vi "Olivia_TrainerLabVIEW.vi"() -> ()   [LabVIEW 2021]
uses:
  <vilib>/Instr/_visa.llb/VISA Configure Serial Port (Instr).vi
panel:
  out "x/y":dbl
  out "Training String":string
  out "Upload String":string
  in  "Training Data":bool
  in  "Upload":bool
  out "Light Intensity %":dbl(slide) scale=0.0..100.0
  in  "Motor Position":dbl(knob) scale=0.0..180.0 scale format="%^#_3g"
  out "Meter":dbl(knob) scale=0.0..10.0
  out "Status indicator":bool
  out "Boolean 2":bool
  out "Boolean":bool
  out "concatenated string":string
  out "Numeric":i32
  out "return count 3":u32
  out "return count 2":u32
  out "read buffer":string
  out "return count":u32
  out "Motor":string
  out "Sensor":string
  out "Type":string
  out "Name":string
  out "read buffer 3":string
  out "Serial Settings:Number of Bytes at Serial Port 2":u32
  out "read buffer 2":string
  in  "VISA resource name 2":refnum<visa-resource-name>
  out "Value":dbl
  out "Motor":dbl(slide) scale=0.0..180.0
  in  "Done":bool
  in  "Train":bool
  # "View & Train"
  # "Green button that says connected"
  # "help button pops up a help message"
  # "big button to connect - Green light to indicate connection"
  # "move the LED to the top to show connection"
  # "Connect"
  # "Make it go back to this screen when nothing is connected"
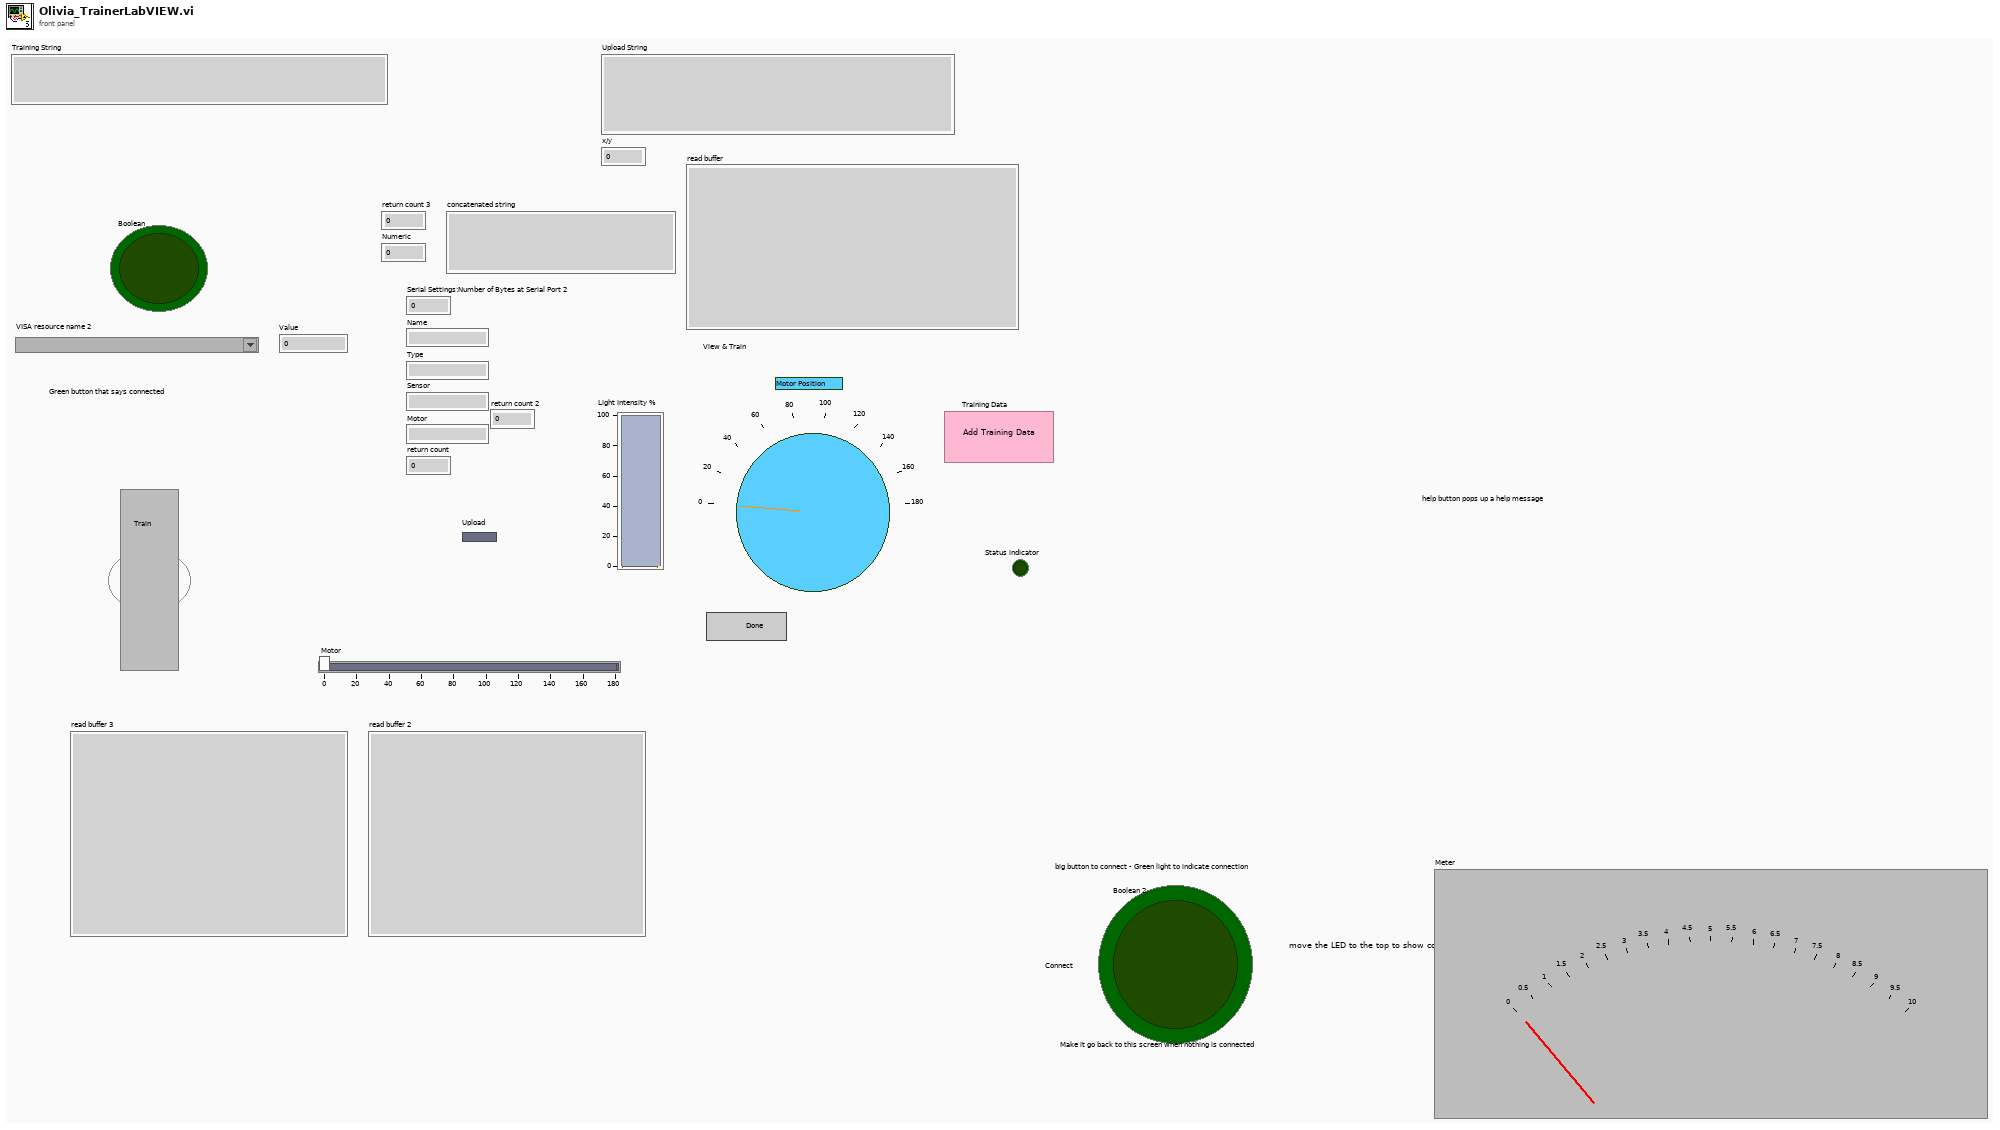
[diagram p1: front panel]
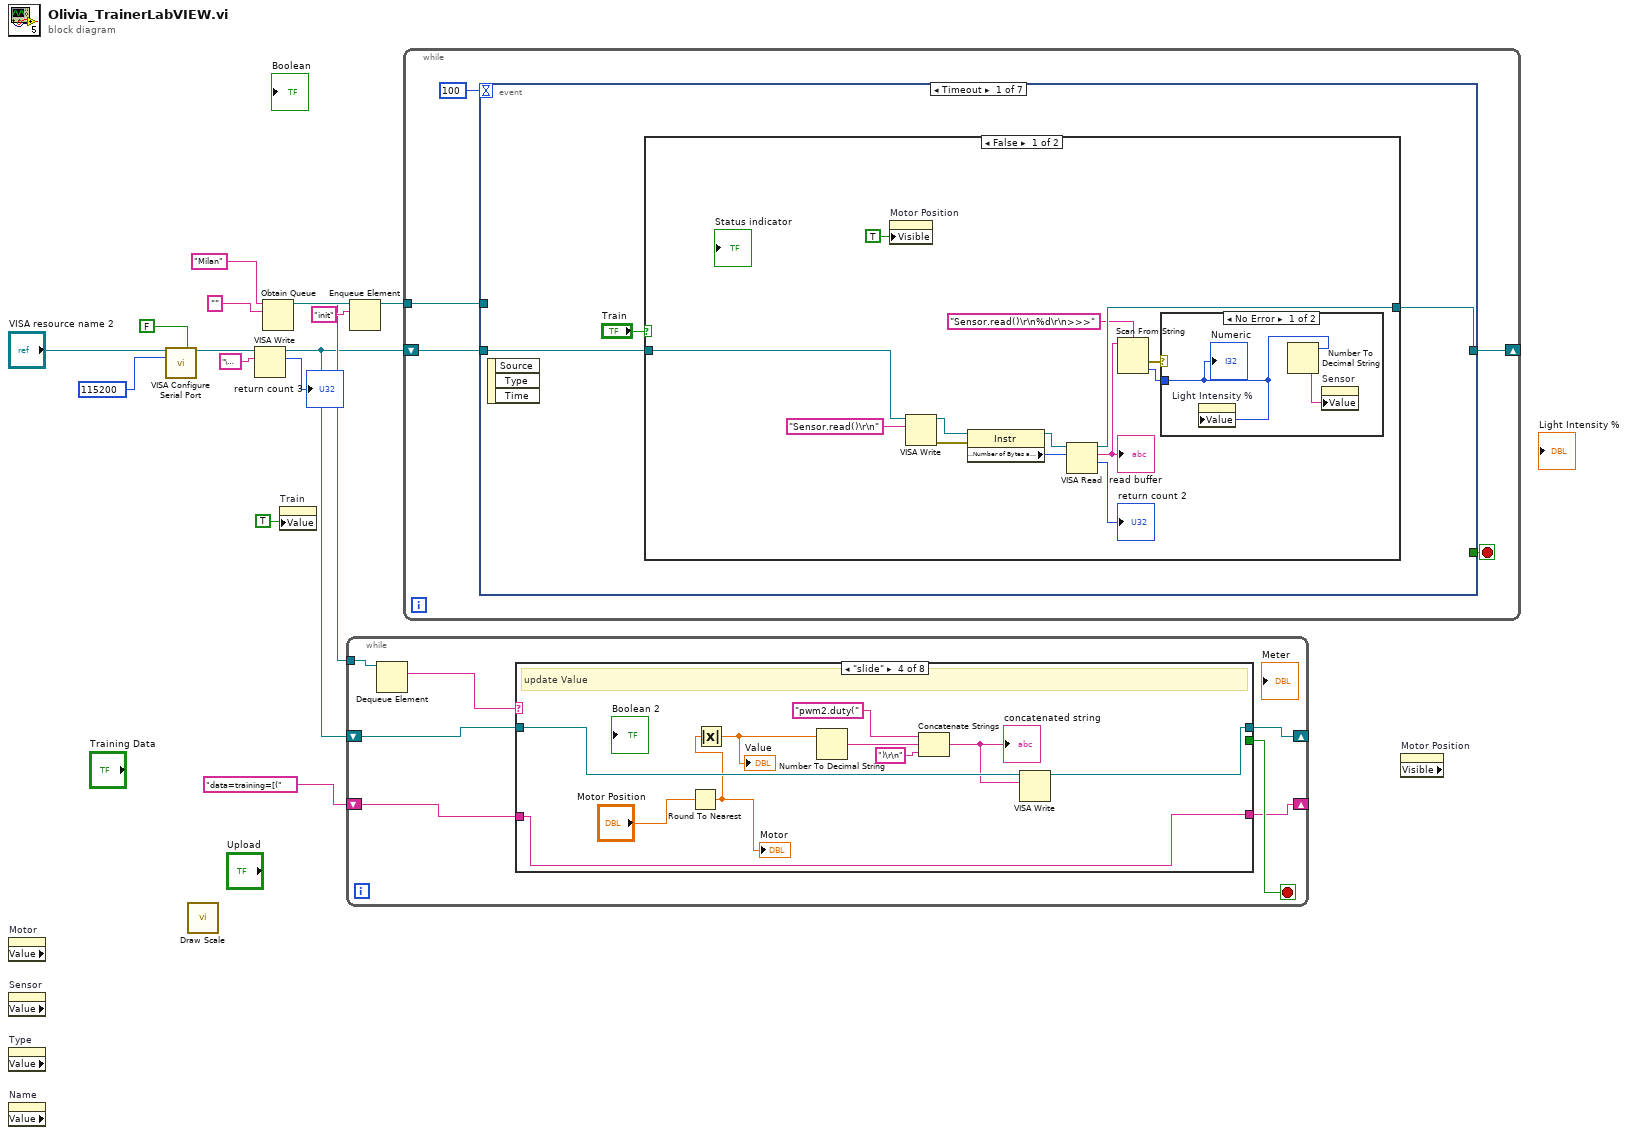
[diagram p0: block diagram]
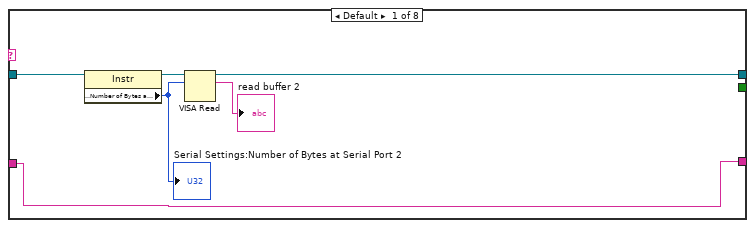
[diagram p2: hidden frame]
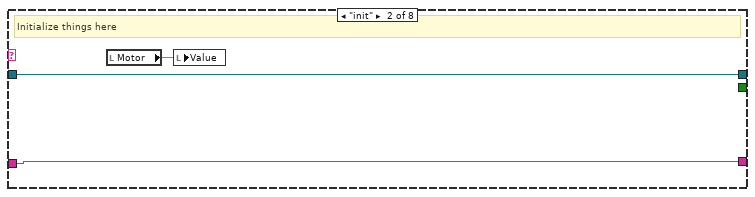
[diagram p3: hidden frame]
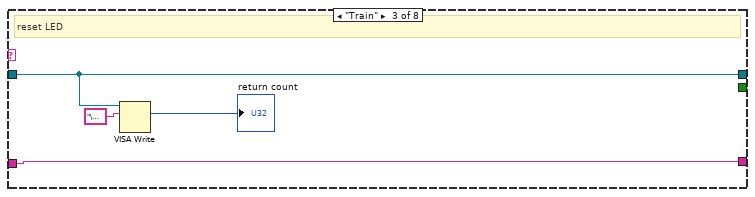
[diagram p4: hidden frame]
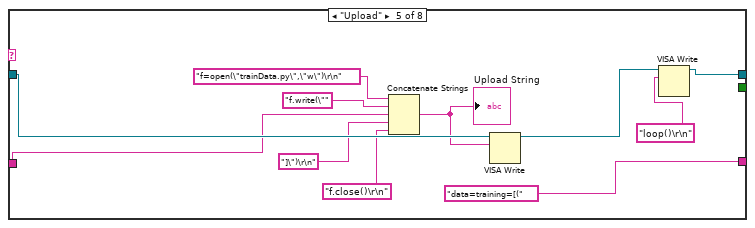
[diagram p5: hidden frame]
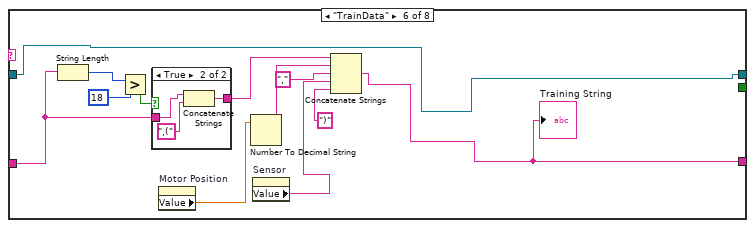
[diagram p6: hidden frame]
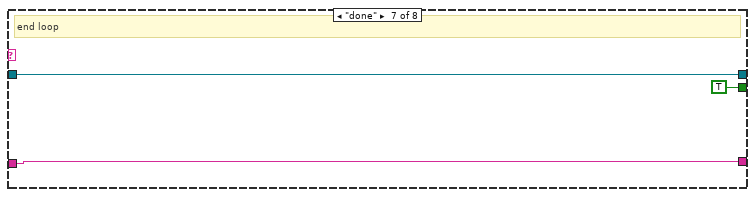
[diagram p8: hidden frame]
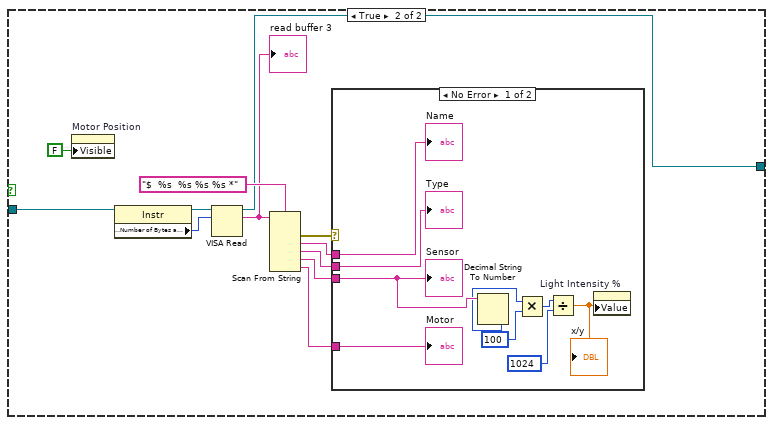
[diagram p11: hidden frame]
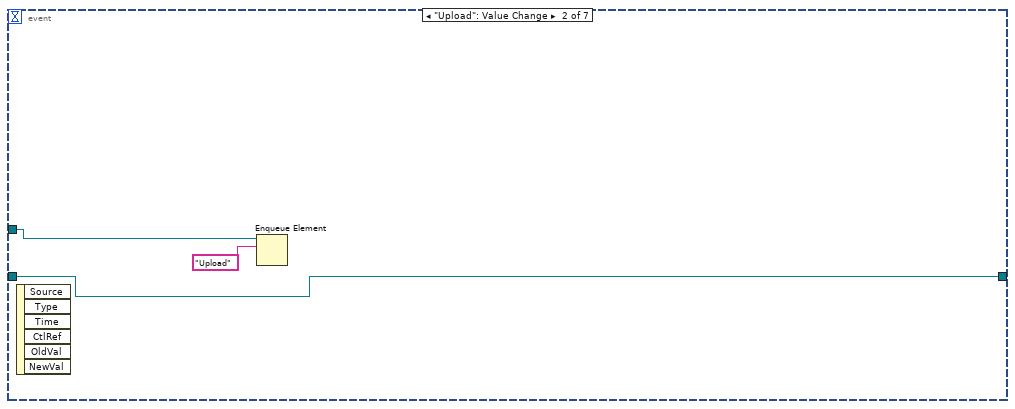
[diagram p13: hidden frame]
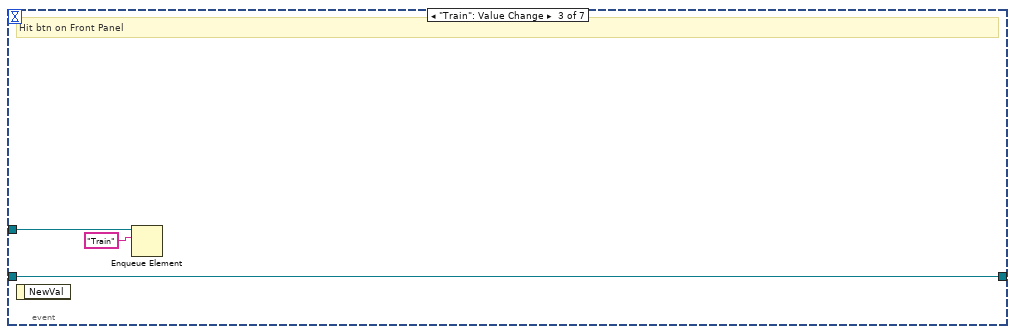
[diagram p14: hidden frame]
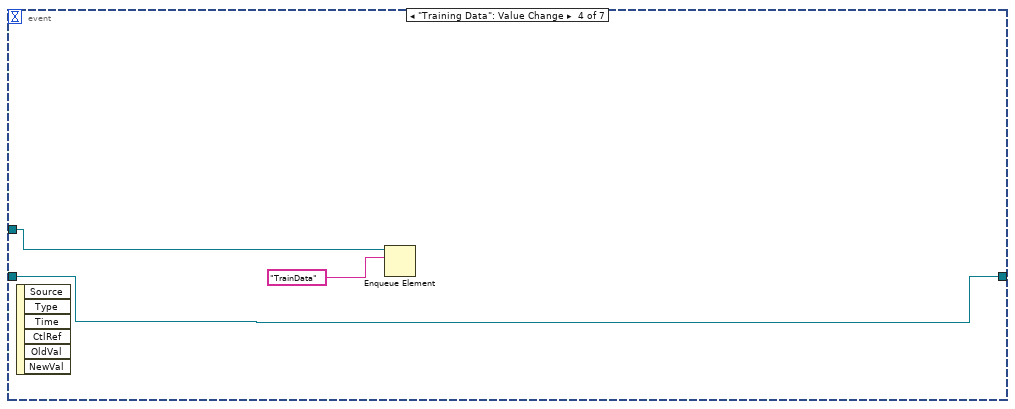
[diagram p15: hidden frame]
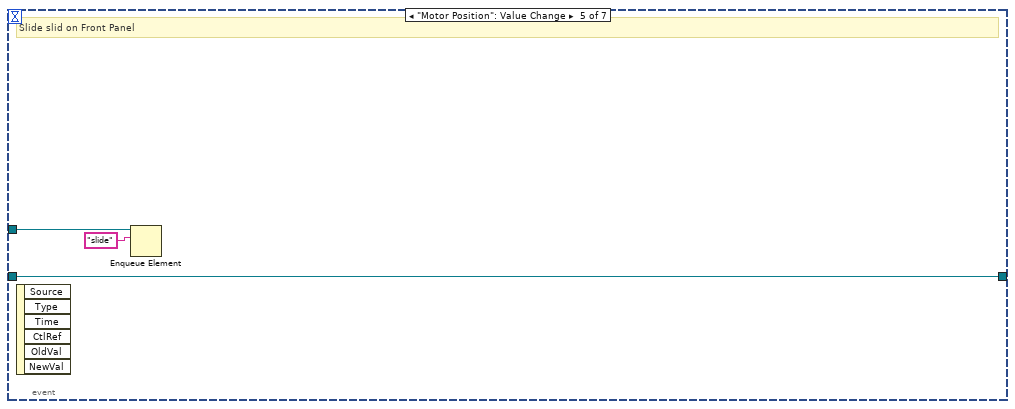
[diagram p16: hidden frame]
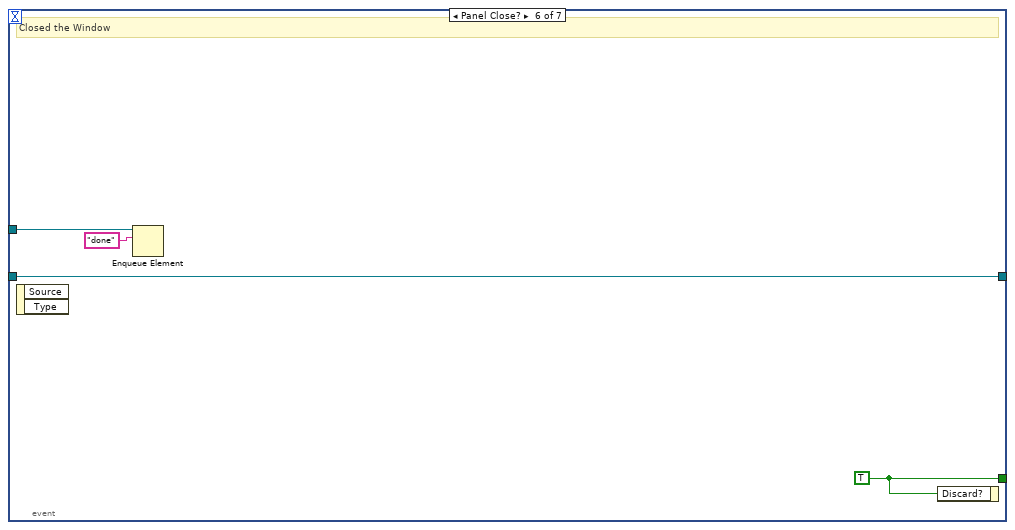
[diagram p17: hidden frame]
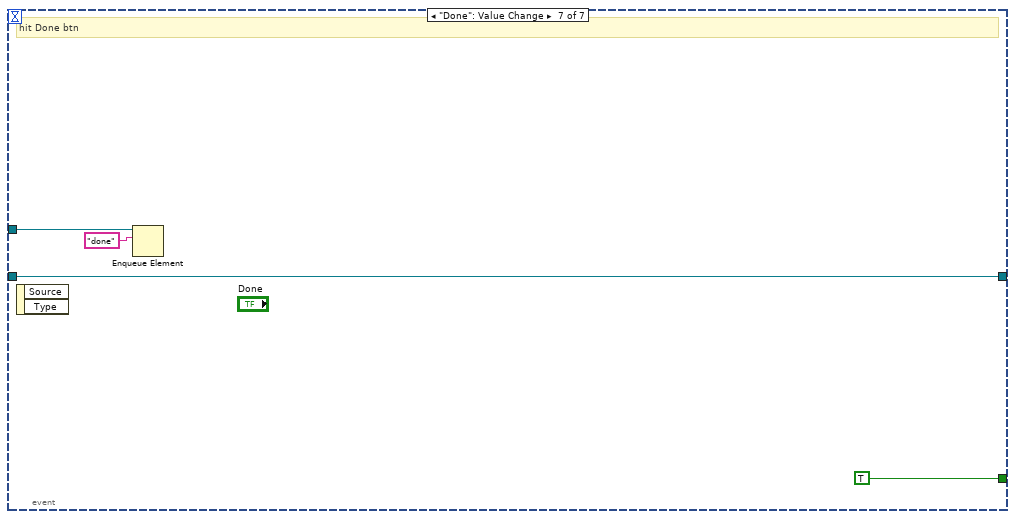
[diagram p18: hidden frame]
diagram:
  n1 = property on="Motor" class="Str" props=["Value"]() -> ()  [unwired: 2 in, 3 out]
  n2 = property on="Sensor" class="Str" props=["Value"]() -> ()  [unwired: 2 in, 3 out]
  n3 = property on="Type" class="Str" props=["Value"]() -> ()  [unwired: 2 in, 3 out]
  n4 = property on="Name" class="Str" props=["Value"]() -> ()  [unwired: 2 in, 3 out]
  n5 = call-poly "VISA Configure Serial Port"("VISA resource name"="VISA resource name 2", "Enable Termination\nChar (T)"=FALSE ("Enable Termination\nChar (T)"), "baud rate (9600)"=u32 115200) -> ("VISA resource name out"=w6:refnum<visa-resource-name>)  [unwired: 11 in, 1 out]
  n6 = call <vilib>:"Draw Scale.vi"() -> ()  [unwired: 11 in, 1 out]
  n7 = VISA Write(VISA resource name=w6, write buffer="\u0004") -> (VISA resource name out=w4:refnum<visa-resource-name>, return count=→"return count 3":u32)  [unwired: 1 in, 1 out]
  n8 = Obtain Queue(name (unnamed)="Milan", element data type="") -> (queue out=w14:refnum<queue>)  [unwired: 3 in, 2 out]
  n9 = property on="Train" class="Bool (strict)"("Value"=TRUE ("Train")) -> ()  [unwired: 2 in, 2 out]
  n10 = Enqueue Element(queue=w14, element="init") -> (queue out=w10:refnum<queue>)  [unwired: 2 in, 2 out]
  n11 = while {
    tunnel: w10 -> [w21]
    shift-right: [w17] -> _
    shift-left: w4 -> [w18]
    shift-right: [w15] -> _
    shift-left: "data=training=[(" -> [w16]
    stop <- w19 stop-if-true
    n12 = Dequeue Element(queue=w21) -> (element=w20:string)  [unwired: 2 in, 3 out]
    n13 = case shown="\"slide\"" w20 {
      tunnel: [_ _ _ _ _ _ TRUE ("Discard?") _] -> w19
      tunnel: w18 -> [w24 w29 w34 w44 w55 w63 w73 w76]
      tunnel: [w23 w29 w34 w39 w46 w63 w73 w76] -> w17
      tunnel: w16 -> [w22 w28 w31 w35 w52 w58 w72 w75]
      tunnel: [w22 w28 w31 w35 "data=training=[(" w56 w72 w75] -> w15
      frame Default {
        n14 = property class="Instr"(reference=w24) -> (reference out=w25:refnum<visa-resource-name>, "Serial Settings:Number of Bytes at Serial Port"=w26:u32)  [unwired: 1 in, 1 out]
        "Serial Settings:Number of Bytes at Serial Port 2" <- w26
        n15 = VISA Read(VISA resource name=w25, byte count=w26) -> (VISA resource name out=w23:refnum<visa-resource-name>, read buffer=→"read buffer 2":string)  [unwired: 1 in, 2 out]
      }
      frame "init" {
        # "Initialize things here"
        n16 = local read "Motor"() -> (w30:dbl)
        n17 = local write "Value"(w30) -> ()
      }
      frame "Train" {
        # "reset LED"
        n18 = VISA Write(VISA resource name=w34, write buffer="\u0003") -> (return count=→"return count":u32)  [unwired: 1 in, 2 out]
      }
      frame "slide" {
        # "update Value"
        n19 = Round To Nearest(number="Motor Position") -> (nearest integer value=w36:dbl)
        "Motor" <- w36
        n20 = Absolute Value(x=w36) -> (abs(x)=w38:dbl)
        "Value" <- w38
        n21 = Number To Decimal String(number=w38) -> (decimal integer string=w42:string)  [unwired: 1 in]
        n22 = Concatenate Strings("pwm2.duty(", w42, ")\r\n" ("string")) -> (w40:string)
        "concatenated string" <- w40
        n23 = VISA Write(VISA resource name=w44, write buffer=w40) -> (VISA resource name out=w39:refnum<visa-resource-name>)  [unwired: 1 in, 2 out]
      }
      frame "Upload" {
        n24 = Concatenate Strings("f=open(\"trainData.py\",\"w\")\r\n" ("string"), "f.write(\"" ("string"), w52, "]\")\r\n" ("string"), "f.close()\r\n" ("string")) -> (w49:string)
        "Upload String" <- w49
        n25 = VISA Write(VISA resource name=w55, write buffer=w49) -> (VISA resource name out=w47:refnum<visa-resource-name>)  [unwired: 1 in, 2 out]
        n26 = VISA Write(VISA resource name=w47, write buffer="loop()\r\n") -> (VISA resource name out=w46:refnum<visa-resource-name>)  [unwired: 1 in, 2 out]
      }
      frame "TrainData" {
        n27 = String Length(string=w58) -> (length=w62:i32)
        n28 = Greater?(x=w62, y=18) -> (0:w60:bool)
        n29 = case shown="True" w60 {
          tunnel: w58 -> [w68 w70]
          tunnel: [w68 w69] -> w59
          frame False {
          }
          frame True {
            n30 = Concatenate Strings(w70, ",(" ("string")) -> (w69:string)
          }
        }
        n31 = property on="Motor Position" class="Knob (strict)"() -> ("Value"=w67:dbl)  [unwired: 2 in, 2 out]
        n32 = Number To Decimal String(number=w67) -> (decimal integer string=w66:string)  [unwired: 1 in]
        n33 = property on="Sensor" class="Str"() -> ("Value"=w57:string)  [unwired: 2 in, 2 out]
        n34 = Concatenate Strings(w59, w66, "," ("string"), w57, ")" ("string")) -> (w56:string)
        "Training String" <- w56
      }
      frame "done" {
        # "end loop"
      }
      frame "" {
      }
    }
  }
  n35 = while {
    tunnel: w10 -> [w81]
    shift-right: [w78] -> _
    shift-left: w4 -> [w79]
    stop <- w80 stop-if-true
    n36 = event shown="[0] Timeout" {
      selector: _ -> [_ _ _ _ _ _ _]
      dyn-events: _ -> [_ _ _ _ _ _ _]
      timeout: 100 -> [_ _ _ _ _ _ _]
      tunnel: w81 -> [_ w123 w125 w128 w131 w135 w139]
      tunnel: [_ _ _ _ _ w134 TRUE ("Discard?")] -> w80
      tunnel: w79 -> [w82 w121 w124 w127 w130 w133 w137]
      tunnel: [w83 w121 w124 w127 w130 w133 w137] -> w78
      event Timeout {
        n37 = event-data() -> ()  [unwired: 1 in, 3 out]
        n38 = case shown="False" "Train" {
          tunnel: w82 -> [w97 w102]
          tunnel: [w92 w104] -> w83
          frame False {
            n39 = property on="Motor Position" class="Knob (strict)"("Visible"=TRUE) -> ()  [unwired: 2 in, 2 out]
            n40 = VISA Write(VISA resource name=w97, write buffer="Sensor.read()\r\n") -> (VISA resource name out=w95:refnum<visa-resource-name>, error out=w90:errorcluster)  [unwired: 1 in, 1 out]
            n41 = property class="Instr"(reference=w95, error in=w90) -> (reference out=w94:refnum<visa-resource-name>, "Serial Settings:Number of Bytes at Serial Port"=w93:u32)  [unwired: 1 out]
            n42 = VISA Read(VISA resource name=w94, byte count=w93) -> (VISA resource name out=w92:refnum<visa-resource-name>, read buffer=w86:string, return count=→"return count 2":u32)  [unwired: 1 in, 1 out]
            "read buffer" <- w86
            n43 = Scan From String(format string="Sensor.read()\r\n%d\r\n>>>", input string=w86) -> (error out=w89:errorcluster, output 1=w88:i32)  [unwired: 3 in, 2 out]
            n44 = case shown="No Error" w89 {
              tunnel: w88 -> [w99 _]
              frame No Error {
                n45 = property on="Light Intensity %" class="Slide (strict)"("Value"=w99) -> ()  [unwired: 2 in, 2 out]
                n46 = Number To Decimal String(number=w99) -> (decimal integer string=w98:string)  [unwired: 1 in]
                n47 = property on="Sensor" class="Str"("Value"=w98) -> ()  [unwired: 2 in, 2 out]
                "Numeric" <- w99
              }
              frame Error {
              }
            }
          }
          frame True {
            n48 = property on="Motor Position" class="Knob (strict)"("Visible"=FALSE) -> ()  [unwired: 2 in, 2 out]
            n49 = property class="Instr"(reference=w102) -> (reference out=w101:refnum<visa-resource-name>, "Serial Settings:Number of Bytes at Serial Port"=w103:u32)  [unwired: 1 in, 1 out]
            n50 = VISA Read(VISA resource name=w101, byte count=w103) -> (VISA resource name out=w104:refnum<visa-resource-name>, read buffer=w105:string)  [unwired: 1 in, 2 out]
            "read buffer 3" <- w105
            n51 = Scan From String(format string="$  %s  %s %s %s *", input string=w105) -> (error out=w111:errorcluster, output 1=w107:string, output 2=w108:string, output 3=w109:string, output 4=w110:string)  [unwired: 6 in, 2 out]
            n52 = case shown="No Error" w111 {
              tunnel: w107 -> [w120 _]
              tunnel: w108 -> [w119 _]
              tunnel: w109 -> [w117 _]
              tunnel: w110 -> [w118 _]
              frame No Error {
                n53 = Decimal String To Number(string=w117) -> (number=w112:i32)  [unwired: 2 in, 1 out]
                n54 = Multiply(x=w112, y=100 ("value")) -> (x*y=w115:i32)
                n55 = Divide(x=w115, y=1024 ("value")) -> (x/y=w113:dbl)
                "x/y" <- w113
                n56 = property on="Light Intensity %" class="Slide (strict)"("Value"=w113) -> ()  [unwired: 2 in, 2 out]
                "Name" <- w120
                "Type" <- w119
                "Sensor" <- w117
                "Motor" <- w118
              }
              frame Error {
              }
            }
          }
        }
      }
      event "Upload": Value Change {
        n57 = event-data() -> ()  [unwired: 1 in, 6 out]
        n58 = Enqueue Element(queue=w123, element="Upload") -> ()  [unwired: 2 in, 3 out]
      }
      event "Train": Value Change {
        # "Hit btn on Front Panel"
        n59 = event-data() -> ()  [unwired: 1 in, 1 out]
        n60 = Enqueue Element(queue=w125, element="Train") -> ()  [unwired: 2 in, 3 out]
      }
      event "Training Data": Value Change {
        n61 = event-data() -> ()  [unwired: 1 in, 6 out]
        n62 = Enqueue Element(queue=w128, element="TrainData") -> ()  [unwired: 2 in, 3 out]
      }
      event "Motor Position": Value Change {
        # "Slide slid on Front Panel"
        n63 = event-data() -> ()  [unwired: 1 in, 6 out]
        n64 = Enqueue Element(queue=w131, element="slide") -> ()  [unwired: 2 in, 3 out]
      }
      event Panel Close? {
        w134 = TRUE ("Discard?")
        # "Closed the Window"
        n65 = event-data() -> ()  [unwired: 1 in, 2 out]
        n66 = Enqueue Element(queue=w135, element="done") -> ()  [unwired: 2 in, 3 out]
        n67 = event-data("Discard?"=w134) -> ()  [unwired: 1 in, 1 out]
      }
      event "Done": Value Change {
        # "hit Done btn"
        n68 = event-data() -> ()  [unwired: 1 in, 2 out]
        n69 = Enqueue Element(queue=w139, element="done") -> ()  [unwired: 2 in, 3 out]
      }
    }
  }
  n70 = property on="Motor Position" class="Knob (strict)" props=["Visible"]() -> ()  [unwired: 2 in, 3 out]
